vi "Tegam4040 - Read SN.vi"(0 "VISA TEGAM 4040A":refnum<visa-resource-name>, 11 "error in (no error)":errorcluster) -> (6 "Serial Number":string, 15 "error out":errorcluster)   [LabVIEW 2010]
doc: "A 32-bit field reserved for the board’s serial number. The value\n0xFFFFFFFF is reserved."
panel:
  out "VISA resource name out":refnum<visa-resource-name>
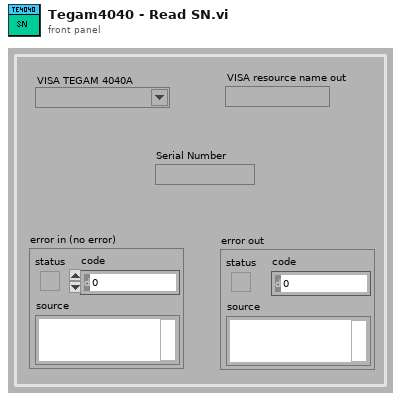
[diagram p1: front panel]
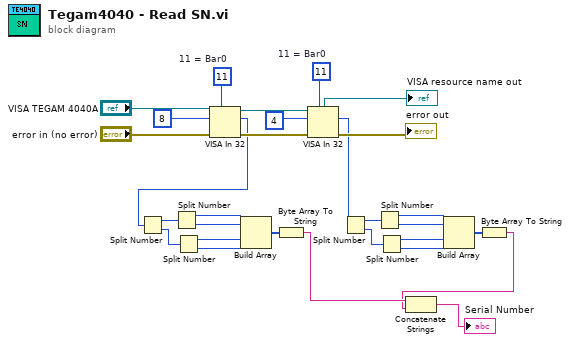
[diagram p0: block diagram]
diagram:
  w22 = u16 11  # 11 = Bar0
  w29 = u16 11  # 11 = Bar0
  n1 = VISA In 32(7:w29, 8:"error in (no error)", 10:u32 8 ("offset (0)"), 11:"VISA TEGAM 4040A") -> (0:w24:errorcluster, 2:w12:u32, 3:w25:refnum<visa-resource-name>)
  n2 = Split Number(x=w12) -> (hi(x)=w19:u16, lo(x)=w18:u16)
  n3 = Split Number(x=w19) -> (hi(x)=w17:u8, lo(x)=w16:u8)
  n4 = Split Number(x=w18) -> (hi(x)=w15:u8, lo(x)=w14:u8)
  n5 = Build Array(w17, w16, w15, w14) -> (w13:u8[])
  n6 = Byte Array To String(unsigned byte array=w13) -> (string=w3:string)
  n7 = VISA In 32(7:w22, 8:w24, 10:u32 4 ("offset (0)"), 11:w25) -> (0:→"error out":errorcluster, 2:w4:u32, 3:→"VISA resource name out":refnum<visa-resource-name>)
  n8 = Split Number(x=w4) -> (hi(x)=w11:u16, lo(x)=w10:u16)
  n9 = Split Number(x=w11) -> (hi(x)=w9:u8, lo(x)=w8:u8)
  n10 = Split Number(x=w10) -> (hi(x)=w7:u8, lo(x)=w6:u8)
  n11 = Build Array(w9, w8, w7, w6) -> (w5:u8[])
  n12 = Byte Array To String(unsigned byte array=w5) -> (string=w2:string)
  n13 = Concatenate Strings(w3, w2) -> (→"Serial Number":string)
